vi "Calculate RPM v3.vi"(9 "Which Formula":T1=enum."Brian", 10 "Basket":T2=enum."Top", 11 "Distance to Target (feet)":dbl=10.0) -> (1 "Calculation Failed":bool, 2 "Calculated initial velocity (m/s)":dbl, 3 "RPM":dbl=1000.0)   [LabVIEW 2012]
uses:
  BasketType.ctl
  FormulaChoose.ctl
  Robot Global Data.vi
  <vilib>/gmath/NI_Gmath.lvlib
panel:
  in  "RPM Bottom":dbl[](array[numeric])=[1000.0, 1100.0, 950.0, 1000.0, 950.0, 1100.0]
  in  "Distance (feet) Bottom":dbl[](array[numeric])=[10.0, 12.0, 13.0, 15.0, 16.0, 17.0]
  in  "RPM Left/Right":dbl[](array[numeric])=[1000.0, 1100.0, 950.0, 1000.0, 950.0, 1100.0]
  in  "Distance (feet) Left/Right":dbl[](array[numeric])=[10.0, 12.0, 13.0, 15.0, 16.0, 17.0]
  in  "RPM Top":dbl[](array[numeric])=[1000.0, 1100.0, 950.0, 1000.0, 950.0, 1100.0]
  in  "Distance (feet) Top":dbl[](array[numeric])=[10.0, 12.0, 13.0, 15.0, 16.0, 17.0]
  # "Data Formula"
  # "Top"
  # "Left/Right"
  # "Bottom"
  # "Brian Formula"
  # "Main"
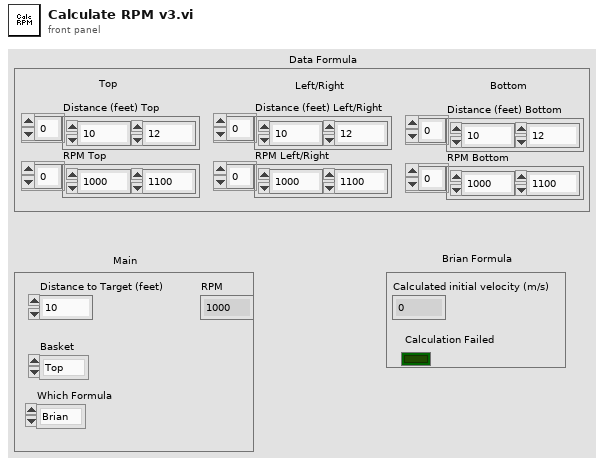
[diagram p1: front panel]
types:
  T1 = typedef "FormulaChoose.ctl" = enum16{"None", "Brian", "Jeremy", "Steven", "Data Based"}
  T2 = typedef "BasketType.ctl" = enum16{"Left", "Bottom", "Right", "Top"}
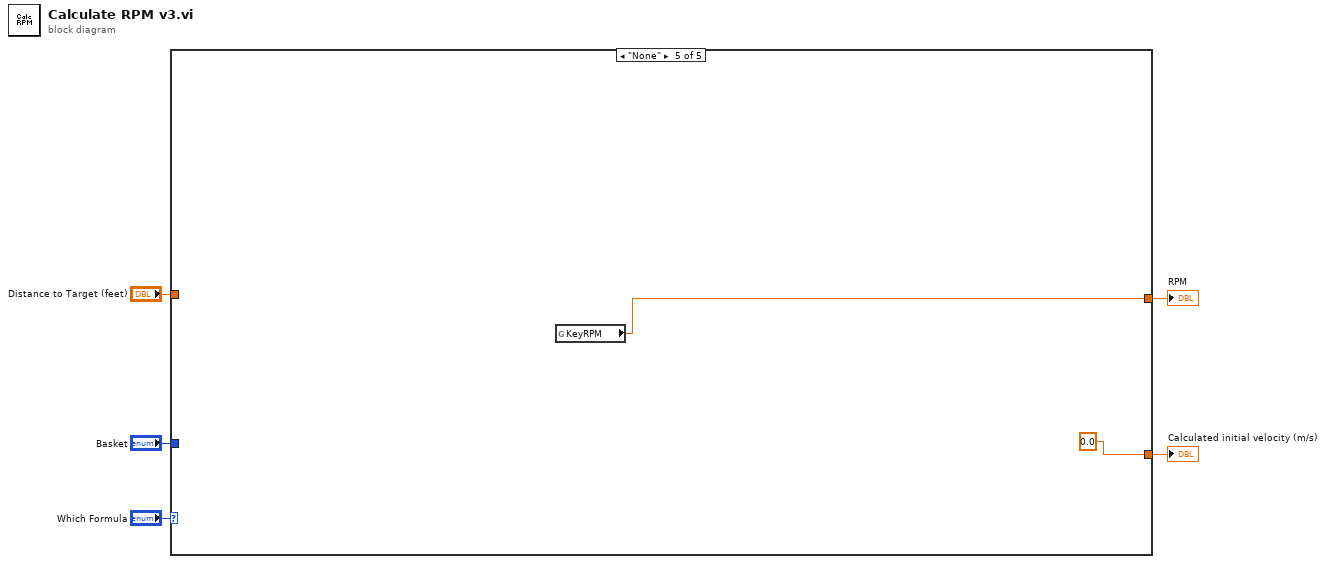
[diagram p0: block diagram]
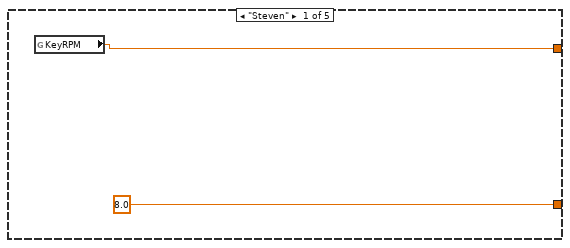
[diagram p2: hidden frame]
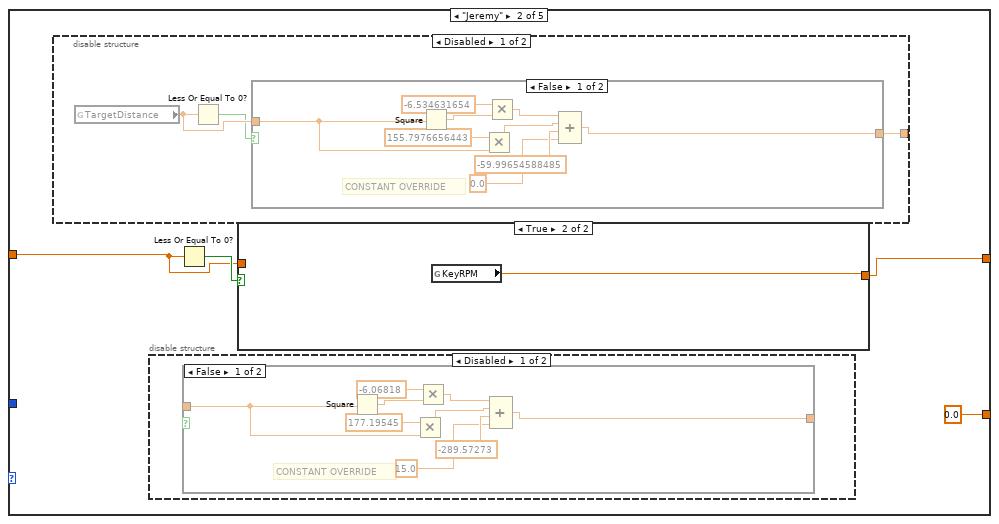
[diagram p3: hidden frame]
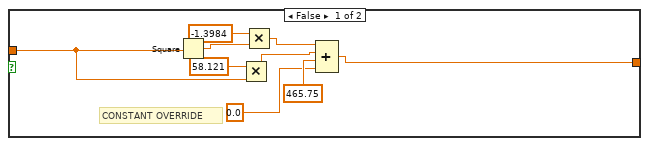
[diagram p4: hidden frame]
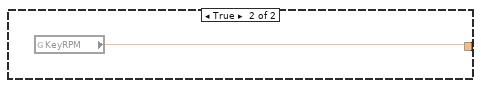
[diagram p5: hidden frame]
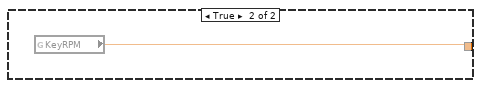
[diagram p7: hidden frame]
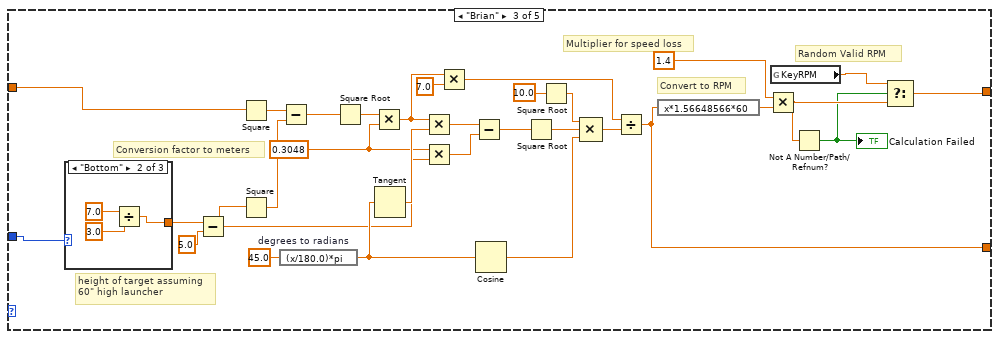
[diagram p9: hidden frame]
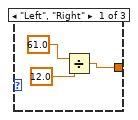
[diagram p10: hidden frame]
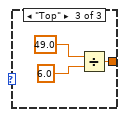
[diagram p11: hidden frame]
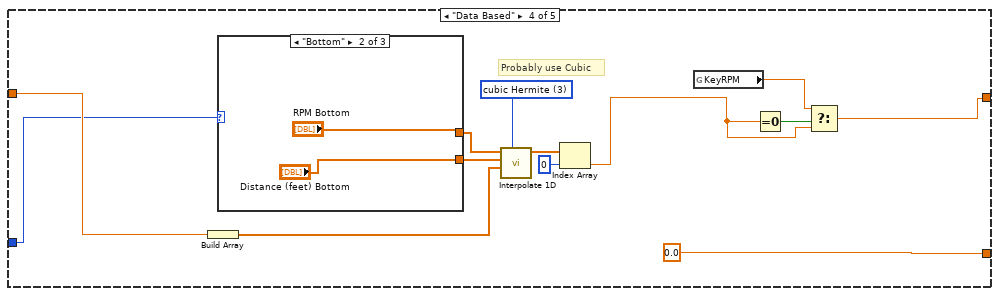
[diagram p12: hidden frame]
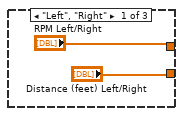
[diagram p13: hidden frame]
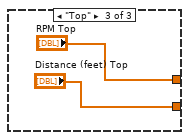
[diagram p14: hidden frame]
diagram:
  n1 = case shown="\"None\"" "Which Formula" {
    tunnel: "Distance to Target (feet)" -> [_ w8 w53 w97 _]
    tunnel: [w6 w9 w52 w86 w105] -> w4
    tunnel: [8.0 0.0 w51 0.0 0.0] -> w3
    tunnel: "Basket" -> [_ _ w48 w90 _]
    frame "Steven" {
      n2 = global read "Robot Global Data.vi" "KeyRPM"() -> (w6:dbl)
    }
    frame "Jeremy" {
      n3 = disable-structure shown="Disabled" {
        disable-tunnel: [w22 _] -> _
        frame Disabled {
          n4 = global read "Robot Global Data.vi" "TargetDistance"() -> (w24:dbl)
          n5 = Less Or Equal To 0?(x=w24) -> (x <= 0?=w23:bool)
          n6 = case shown="False" w23 {
            tunnel: [w25 w34] -> w22
            tunnel: w24 -> [w28 _]
            frame False {
              # "CONSTANT OVERRIDE"
              n7 = Square(x=w28) -> (x^2=w33:dbl)
              n8 = Multiply(x=155.7976656443, y=w28) -> (x*y=w31:dbl)
              n9 = Multiply(x=-6.534631654, y=w33) -> (x*y=w32:dbl)
              n10 = Compound Arithmetic op=ADD(w32, w31, -59.99654588485 ("value"), 0.0 ("value")) -> (w25:dbl)
            }
            frame True {
              n11 = global read "Robot Global Data.vi" "KeyRPM"() -> (w34:dbl)
            }
          }
        }
        frame Enabled {
        }
      }
      n12 = disable-structure shown="Disabled" {
        frame Disabled {
          n13 = case shown="False" {
            selector: _ -> [_ _]
            tunnel: [w35 w44] -> _
            tunnel: _ -> [w38 _]
            frame False {
              # "CONSTANT OVERRIDE"
              n14 = Square(x=w38) -> (x^2=w43:dbl)
              n15 = Multiply(x=177.19545, y=w38) -> (x*y=w41:dbl)
              n16 = Multiply(x=-6.06818, y=w43) -> (x*y=w42:dbl)
              n17 = Compound Arithmetic op=ADD(w42, w41, -289.57273 ("value"), 15.0 ("value")) -> (w35:dbl)
            }
            frame True {
              n18 = global read "Robot Global Data.vi" "KeyRPM"() -> (w44:dbl)
            }
          }
        }
        frame Enabled {
        }
      }
      n19 = Less Or Equal To 0?(x=w8) -> (x <= 0?=w10:bool)
      n20 = case shown="True" w10 {
        tunnel: [w12 w21] -> w9
        tunnel: w8 -> [w15 _]
        frame False {
          # "CONSTANT OVERRIDE"
          n21 = Square(x=w15) -> (x^2=w20:dbl)
          n22 = Multiply(x=58.121, y=w15) -> (x*y=w18:dbl)
          n23 = Multiply(x=-1.3984, y=w20) -> (x*y=w19:dbl)
          n24 = Compound Arithmetic op=ADD(w19, w18, 465.75 ("value"), 0.0 ("value")) -> (w12:dbl)
        }
        frame True {
          n25 = global read "Robot Global Data.vi" "KeyRPM"() -> (w21:dbl)
        }
      }
    }
    frame "Brian" {
      w61 = 0.3048 ("y")
      # "height of target assuming\n60\" high launcher"
      # "Random Valid RPM"
      # "Multiplier for speed loss"
      # "Convert to RPM"
      # "Conversion factor to meters"
      n26 = case shown="\"Bottom\"" w48 {
        tunnel: [w76 w79 w82] -> w50
        frame "Left", "Right" {
          n27 = Divide(x=61.0, y=12.0) -> (x/y=w76:dbl)
        }
        frame "Bottom" {
          n28 = Divide(x=7.0, y=3.0) -> (x/y=w79:dbl)
        }
        frame "Top" {
          n29 = Divide(x=49.0, y=6.0) -> (x/y=w82:dbl)
        }
      }
      n30 = Subtract(x=w50, y=5.0) -> (x-y=w46:dbl)
      n31 = Square(x=w53) -> (x^2=w59:dbl)
      n32 = Square(x=w46) -> (x^2=w58:dbl)
      n33 = expression code="(x/180.0)*pi" "degrees to radians"(45.0 ("Angle (deg)")) -> (w67:dbl)
      n34 = Subtract(x=w59, y=w58) -> (x-y=w57:dbl)
      n35 = Square Root(x=w57) -> (sqrt(x)=w56:dbl)
      n36 = Multiply(x=w56, y=w61) -> (x*y=w62:dbl)
      n37 = Tangent(1:w67) -> (0:w73:dbl)
      n38 = Multiply(x=w62, y=w73) -> (x*y=w72:dbl)
      n39 = Multiply(x=w61, y=w46) -> (x*y=w60:dbl)
      n40 = Multiply(x=w62, y=7.0) -> (x*y=w63:dbl)
      n41 = Subtract(x=w72, y=w60) -> (x-y=w71:dbl)
      n42 = Cosine(x=w67) -> (cos(x)=w69:dbl)
      n43 = Square Root(x=w71) -> (sqrt(x)=w70:dbl)
      n44 = Square Root(x=10.0) -> (sqrt(x)=w74:dbl)
      n45 = Compound Arithmetic op=MULTIPLY(w74, w70, w69) -> (w68:dbl)
      n46 = Divide(x=w63, y=w68) -> (x/y=w51:dbl)
      n47 = expression code="x*1.56648566*60"(w51) -> (w65:dbl)
      n48 = Multiply(x=1.4, y=w65) -> (x*y=w55:dbl)
      n49 = global read "Robot Global Data.vi" "KeyRPM"() -> (w45:dbl)
      n50 = Not A Number/Path/Refnum?(number/path/refnum=w55) -> (NaN/Path/Refnum?=w54:bool)
      "Calculation Failed" <- w54
      n51 = Select(t=w45, s=w54, f=w55) -> (s? t:f=w52:dbl)
    }
    frame "Data Based" {
      w89 = 3 items=["nearest", "linear", "spline", "cubic Hermite", "Lagrange"] ("method")
      # "Probably use Cubic"
      n52 = Build Array(w97) -> (w96:dbl[])
      n53 = case shown="\"Bottom\"" w90 {
        tunnel: ["RPM Left/Right" "RPM Bottom" "RPM Top"] -> w92
        tunnel: ["Distance (feet) Left/Right" "Distance (feet) Bottom" "Distance (feet) Top"] -> w91
        frame "Left", "Right" {
        }
        frame "Bottom" {
        }
        frame "Top" {
        }
      }
      n54 = call <vilib>:"Interpolate 1D.vi"("method"=w89, "xi"=w96, "X"=w91, "Y"=w92) -> ("yi"=w95:dbl[])  [unwired: 5 in, 2 out]
      n55 = Index Array(array=w95, index=0) -> (element=w87:dbl)
      n56 = global read "Robot Global Data.vi" "KeyRPM"() -> (w85:dbl)
      n57 = Equal To 0?(x=w87) -> (x = 0?=w88:bool)
      n58 = Select(t=w85, s=w88, f=w87) -> (s? t:f=w86:dbl)
    }
    frame "None" {
      n59 = global read "Robot Global Data.vi" "KeyRPM"() -> (w105:dbl)
    }
  }
  "RPM" <- w4
  "Calculated initial velocity (m/s)" <- w3
